vi "XY Graph Sliced Mean & SDV Plots Event.vi"(8 "Error In":errorcluster, 10 "Mouse Coordinates":T1, 11 "Multiplot XY Graph":T2) -> (0 "Error Out":errorcluster, 1 "Message":string)   [LabVIEW 2021, in "XY Graph Add-Ons.lvlib"]
uses:
  XY Graph Add-Ons.lvlib
  XY Graph Refnum.ctl
  <vilib>/Utility/miscctls.llb/LVPoint32TypeDef.ctl
  Get Plot at Mouse Click (XY Graph)/Get Plot at Mouse Click [AAC].vi
  XY Graph Add Multiplots with Names.vi
  Graphs.lvlib
  Variant/Variant.lvlib
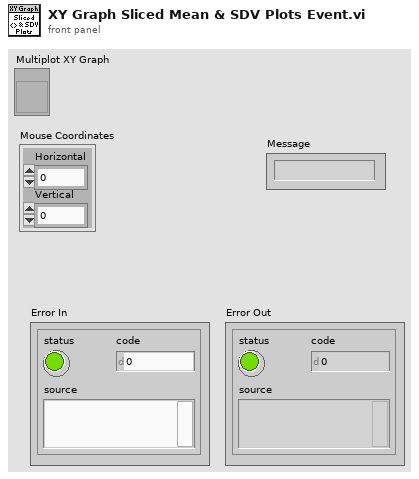
[diagram p1: front panel]
types:
  T1 = typedef "LVPoint32TypeDef.ctl" = cluster{"Horizontal":i32, "Vertical":i32}
  T2 = typedef "XY Graph Add-Ons.lvlib/XY Graph Refnum.ctl" = refnum<vi>
  T3 = typedef "XY Graph Add-Ons.lvlib/XY Graph Slides Mean & SDV Step Definition.ctl" = cluster{"Axis Start":dbl, "Axis Stop":dbl, "# Steps":i32, "Step Size":dbl, "Step Definition":enum32{"# Steps", "Step Size"}, "Upper Percentile":dbl, "Lower Percentile":dbl, "Min # Data Points/Slice":i32, "Output Abscissa Statistics Plots":bool}
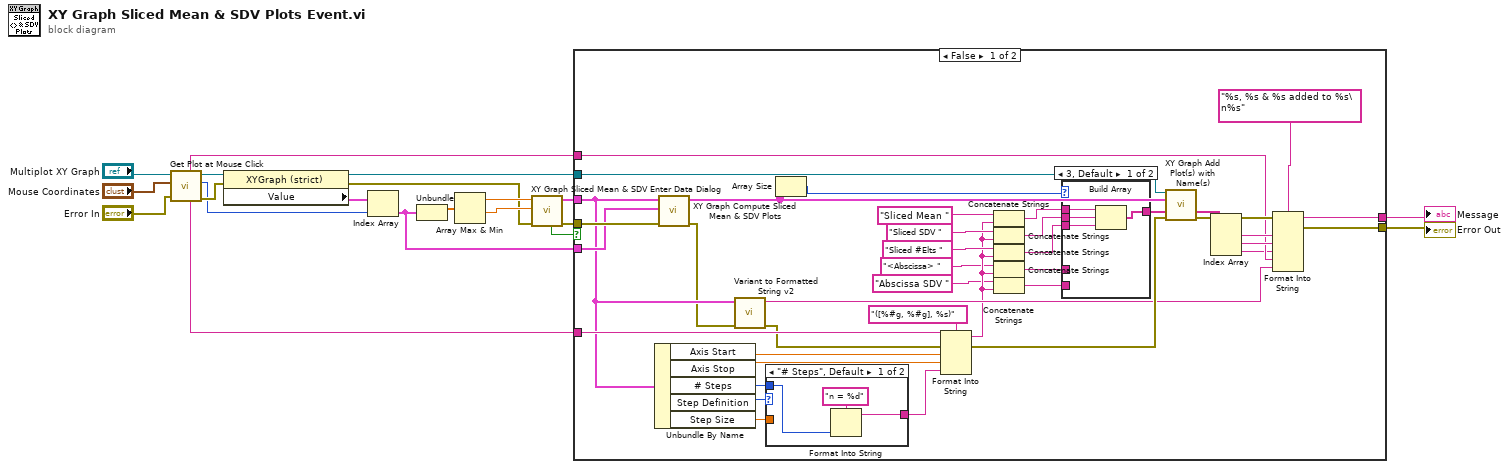
[diagram p0: block diagram]
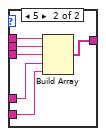
[diagram p2: hidden frame]
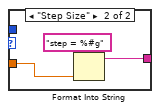
[diagram p3: hidden frame]
diagram:
  n1 = call-poly "Get Plot at Mouse Click.vi"("error in (no error)"="Error In", "Mouse Click Coordinates"="Mouse Coordinates", "XYGraph Ref"="Multiplot XY Graph") -> ("error out"=w18:errorcluster, "Plot at Coordinates"=w16:i32, "XYGraph Ref"=w19:T2, "Plot Name"=w3:string, "Graph Name"=w14:string)  [unwired: 2 in, 2 out]
  n2 = property class="XYGraph (strict)"(reference=w19, error in=w18) -> (reference out=w15:T2, error out=w8:errorcluster, "Value"=w17:cluster{"X Array":dbl[], "Y Array":dbl[]}[])
  n3 = Index Array(array=w17, index=w16) -> (element=w6:cluster{"X Array":dbl[], "Y Array":dbl[]})
  n4 = Unbundle(w6) -> ("X Array"=w11:dbl[])  [unwired: 1 out]
  n5 = Array Max & Min(array=w11) -> (max value=w10:dbl, min value=w9:dbl)  [unwired: 2 out]
  n6 = call "XY Graph Sliced Mean & SDV Enter Data Dialog.vi"("Error In"=w8, "X min"=w9, "X max"=w10) -> ("Error Out"=w7:errorcluster, "Slices Definition"=w5:T3, "Cancelled?"=w4:bool)  [unwired: 6 in]
  n7 = case shown="False" w4 {
    tunnel: w15 -> [w59 _]
    tunnel: w14 -> [w43 _]
    tunnel: [w57 _] -> w13
    tunnel: [w55 w76] -> w12
    tunnel: w7 -> [w54 w76]
    tunnel: w6 -> [w53 _]
    tunnel: w5 -> [w31 _]
    tunnel: w3 -> [w52 _]
    frame False {
      n8 = Unbundle By Name(w31) -> ("Axis Start"=w42:dbl, "Axis Stop"=w41:dbl, "# Steps"=w47:i32, "Step Definition"=w48:enum32{"# Steps", "Step Size"}, "Step Size"=w46:dbl)
      n9 = call "XY Graph Compute Sliced Mean & SDV Plots.vi"("error in (no error)"=w54, "Plot"=w53, "Slices Definition"=w31) -> ("error out"=w21:errorcluster, "Plots"=w28:cluster{"X Array":dbl[], "Y Array":dbl[]}[])  [unwired: 7 in]
      n10 = call "Variant to Formatted String v2.vi"("error in (no error)"=w21, "Anything"=w31) -> ("error out"=w30:errorcluster, "String"=w29:string)  [unwired: 8 in]
      n11 = case shown="\"# Steps\", Default" w48 {
        tunnel: w47 -> [w72 _]
        tunnel: [w70 w74] -> w40
        tunnel: w46 -> [_ w73]
        frame "# Steps", Default {
          n12 = Format Into String(format string="n = %d", w72) -> (resulting string=w70:string)  [unwired: 2 in, 1 out]
        }
        frame "Step Size" {
          n13 = Format Into String(format string="step = %#g", w73) -> (resulting string=w74:string)  [unwired: 2 in, 1 out]
        }
      }
      n14 = Array Size(array=w28) -> (size(s)=w27:i32)
      n15 = Format Into String(format string="([%#g, %#g], %s)", initial string=w52, error in=w30, w42, w41, w40) -> (resulting string=w24:string, error out=w39:errorcluster)
      n16 = Concatenate Strings("Sliced Mean " ("format string"), w24) -> (w35:string)
      n17 = Concatenate Strings("Sliced SDV " ("format string"), w24) -> (w34:string)
      n18 = Concatenate Strings("Sliced #Elts " ("format string"), w24) -> (w33:string)
      n19 = Concatenate Strings("<Abscissa> " ("format string"), w24) -> (w26:string)
      n20 = Concatenate Strings("Abscissa SDV " ("format string"), w24) -> (w25:string)
      n21 = case shown="3, Default" w27 {
        tunnel: [w63 w69] -> w50
        tunnel: w35 -> [w62 w68]
        tunnel: w34 -> [w61 w67]
        tunnel: w33 -> [w60 w66]
        tunnel: w26 -> [_ w65]
        tunnel: w25 -> [_ w64]
        frame 3, Default {
          n22 = Build Array(w62, w61, w60) -> (w63:string[])
        }
        frame 5 {
          n23 = Build Array(w68, w67, w66, w65, w64) -> (w69:string[])
        }
      }
      n24 = call-poly "XY Graph Add Plot(s) with Name(s).vi"("XYGraph in"=w59, "Array of Plots"=w28, "Array of Plot Names (\"Plot\")"=w50, "error in (no error)"=w39) -> ("Added Plot Names"=w49:string[], "error out"=w58:errorcluster)  [unwired: 7 in, 3 out]
      n25 = Index Array(array=w49) -> (element #1=w45:string, element #2=w44:string, element #3=w32:string)  [unwired: 3 in]
      n26 = Format Into String(format string="%s, %s & %s added to %s\n%s", error in=w58, w45, w44, w32, w43, w29) -> (resulting string=w57:string, error out=w55:errorcluster)  [unwired: 1 in]
    }
    frame True {
      # "Cancelled"
    }
  }
  "Error Out" <- w12
  "Message" <- w13
